vi "Post Build VI.vi"() -> ()   [LabVIEW 2013]
panel:
  out "error out":errorcluster
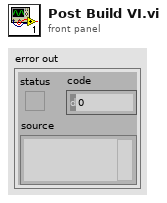
[diagram p1: front panel]
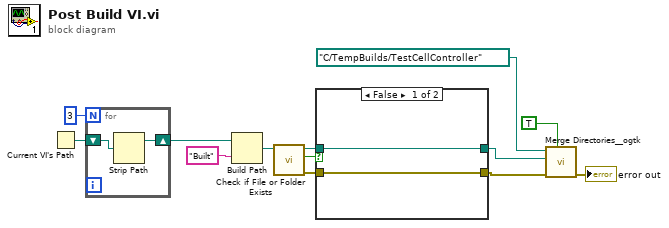
[diagram p0: block diagram]
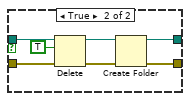
[diagram p2: hidden frame]
diagram:
  n1 = Current VI's Path() -> (path=w13:path)
  n2 = for {
    N: 3 -> [_]
    shift-right: [w14] -> w12
    shift-left: w13 -> [w15]
    n3 = Strip Path(path=w15) -> (stripped path=w14:path)  [unwired: 1 out]
  }
  n4 = Build Path(base path=w12, name or relative path="Built") -> (appended path=w10:path)
  n5 = call <vilib>:"Check if File or Folder Exists.vi"("path"=w10) -> ("error out"=w8:errorcluster, "file or folder exists?"=w9:bool, "dup path"=w7:path)  [unwired: 8 in]
  n6 = case shown="False" w9 {
    tunnel: w8 -> [w16 w24]
    tunnel: w7 -> [w17 w20]
    tunnel: [w16 w23] -> w6
    tunnel: [w17 w22] -> w5
    frame False {
    }
    frame True {
      n7 = Delete(path (use dialog)=w20, entire hierarchy (F)=TRUE, error in=w24) -> (deleted path=w19:path, error out=w21:errorcluster)  [unwired: 2 in, 1 out]
      n8 = Create Folder(path (use dialog)=w19, error in=w21) -> (created path=w22:path, error out=w23:errorcluster)  [unwired: 1 in, 1 out]
    }
  }
  n9 = call <userlib>:"Merge Directories__ogtk.vi"("Delete Source? (FALSE)"=TRUE, "error in (no error)"=w6, "target directory path"=w5, "source directory path"=path "C:/TempBuilds/TestCellController") -> ("error out"=→"error out":errorcluster)  [unwired: 6 in, 1 out]
